vi "Read Long.vi"(11 "GDSII.DataType.Long in":refnum<class "GDSII.DataType.Long.lvclass">) -> (2 "Long":i32[](array[numeric]), 3 "GDSII.DataType.Long out":refnum<class "GDSII.DataType.Long.lvclass">)   [LabVIEW 2019, in "GDSII.DataType.Long.lvclass"]
uses:
  GDSII.DataType.Long.lvclass
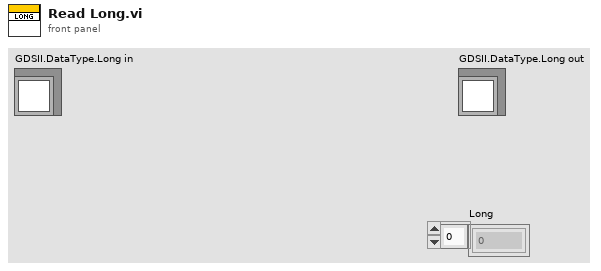
[diagram p1: front panel]
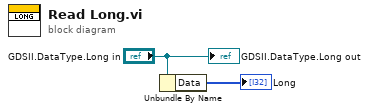
[diagram p0: block diagram]
diagram:
  n1 = Unbundle By Name("GDSII.DataType.Long in") -> ("Data"=→"Long":i32[])
  "GDSII.DataType.Long out" <- "GDSII.DataType.Long in"
